vi "SaveDeviceHeader.vi"(0 "File Refnum in":refnum<file>, 1 "no. of arrays":i32, 3 "Array Lengths":i32, 5 "Filename":string, 7 "Run Number":i32, 9 "Array Titles":string, 11 "error in (no error)":errorcluster, 12 "Temperature":dbl, 13 "Humidity":dbl, 14 "Strip Segment":string) -> (4 "File Refnum out":refnum<file>, 6 "Header string":string, 10 "error out":errorcluster)   [LabVIEW 2018]
uses:
  globals/QC_RunInformation.vi
  globals/QC_MeasurementSetup.vi
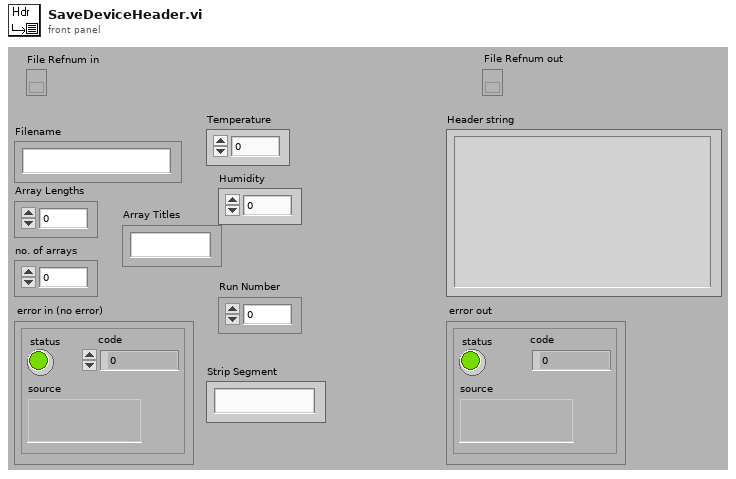
[diagram p1: front panel]
types:
  T1 = cluster{"Institute":string, "Manufacturers":string[], "Devices":string[], "Serialnumbers Lookup DB":string, "Data directory":string, "Backup & screenshot directory":string, "List of known users":string[], "Measurement switch not used":bool, "Measurement Switch":string, "DUT Switch":string}
  T2 = cluster{"Sensor Serial No.:":string, "Wafer Serial No.:":string, "Batch:":string, "Manufacturer:":string, "Device Category:":string, "Database Serial No.:":string, "Date Initiated:":string, "Time Initiated:":string, "Test":string, "Instruments used:":string, "Probeplan used:":string, "End of Run comment:":string, "User:":string}
  T3 = cluster{"Supply":refnum<class "SupplyControl.lvclass">, "LCR":refnum<class "LCRControl.lvclass">, "Initial Voltage [V]":dbl, "Final Voltage [V]":dbl, "Step Size [V]":dbl, "Step Interval [s]":i32, "Number Of Steps":u32, "AC frequency [Hz]":i32, "RC Configuration":u16, "AC amplitude [V]":dbl, "Ramp down steps [V]":dbl, "Ramp down Interval [s]":i32, "Set Current Limit?":bool, "Current Limit [µA]":dbl, "Temperature Readout":enum16{"Read Arduino", "Enter manually"}, "Arduino":refnum<class "ArduinoControl.lvclass">, "Supply Name":string, "LCR Name":string, "V_depletion Limit [V]":dbl, "Switching":refnum<class "Switching.lvclass">, "Matrix used?":bool, "Matrix X Channels":cluster{"Bias Supply / SMU LO":i32, "Bias Supply / SMU HI":i32, "CV Box LO":i32, "CV Box HI":i32, "CV Box LO IN":i32, "CV Box HI IN":i32, "Volt meter LO":i32, "Volt meter HI":i32, "Mux1 C1":i32, "Mux1 C2":i32, "Mux2 C1":i32, "Mux2 C2":i32}}
  T4 = cluster{"Bias Supply":refnum<class "SupplyControl.lvclass">, "SMU":refnum<class "SupplyControl.lvclass">, "LCR":refnum<class "LCRControl.lvclass">, "Probe Card Channels":i32, "Bias Voltage [V]":dbl, "First strip":i32, "Last strip":i32, "Base Voltage [V]":dbl, "Base Ramp Step [V]":dbl, "Base Ramp Interval [ms]":u32, "High Voltage [V]":dbl, "High Ramp Step [V]":dbl, "High Ramp Interval [ms]":u32, "AC frequency [Hz]":i32, "AC amplitude [V]":dbl, "RC Configuration":u16, "Single Needle":bool, "Temperature Readout":enum16{"Read Arduino", "Enter manually"}, "Arduino":refnum<class "ArduinoControl.lvclass">, "Fraction of good strips [%]":dbl, "ProbeStation":refnum<class "ProbeStationControl.lvclass">, "Switching":refnum<class "Switching.lvclass">, "Matrix used?":bool, "Matrix X Channels":cluster{"Bias Supply / SMU LO":i32, "Bias Supply / SMU HI":i32, "CV Box LO":i32, "CV Box HI":i32, "CV Box LO IN":i32, "CV Box HI IN":i32, "Volt meter LO":i32, "Volt meter HI":i32, "Mux1 C1":i32, "Mux1 C2":i32, "Mux2 C1":i32, "Mux2 C2":i32}, "Pinholes Y/N":bool, "Capacitance Y/N":bool, "Resistance Y/N":bool, "Bias Supply Name":string, "SMU Name":string, "LCR Name":string}
  T5 = cluster{"Supply":refnum<class "SupplyControl.lvclass">, "LCR":refnum<class "LCRControl.lvclass">, "Initial Voltage [V]":dbl, "Final Voltage [V]":dbl, "Step Size [V]":dbl, "Step Interval [s]":i32, "Number Of Steps":u32, "AC frequency [Hz]":i32, "RC Configuration":u16, "AC amplitude [V]":dbl, "Ramp down steps [V]":dbl, "Ramp down Interval [s]":i32, "Set Current Limit?":bool, "Current Limit [µA]":dbl, "Temperature Readout":enum16{"Read Arduino", "Enter manually"}, "Arduino":refnum<class "ArduinoControl.lvclass">, "Supply Name":string, "LCR Name":string, "C_is Limit [pF/cm]":dbl, "Switching":refnum<class "Switching.lvclass">, "Matrix used?":bool, "Matrix X Channels":cluster{"Bias Supply / SMU LO":i32, "Bias Supply / SMU HI":i32, "CV Box LO":i32, "CV Box HI":i32, "CV Box LO IN":i32, "CV Box HI IN":i32, "Volt meter LO":i32, "Volt meter HI":i32, "Mux1 C1":i32, "Mux1 C2":i32, "Mux2 C1":i32, "Mux2 C2":i32}}
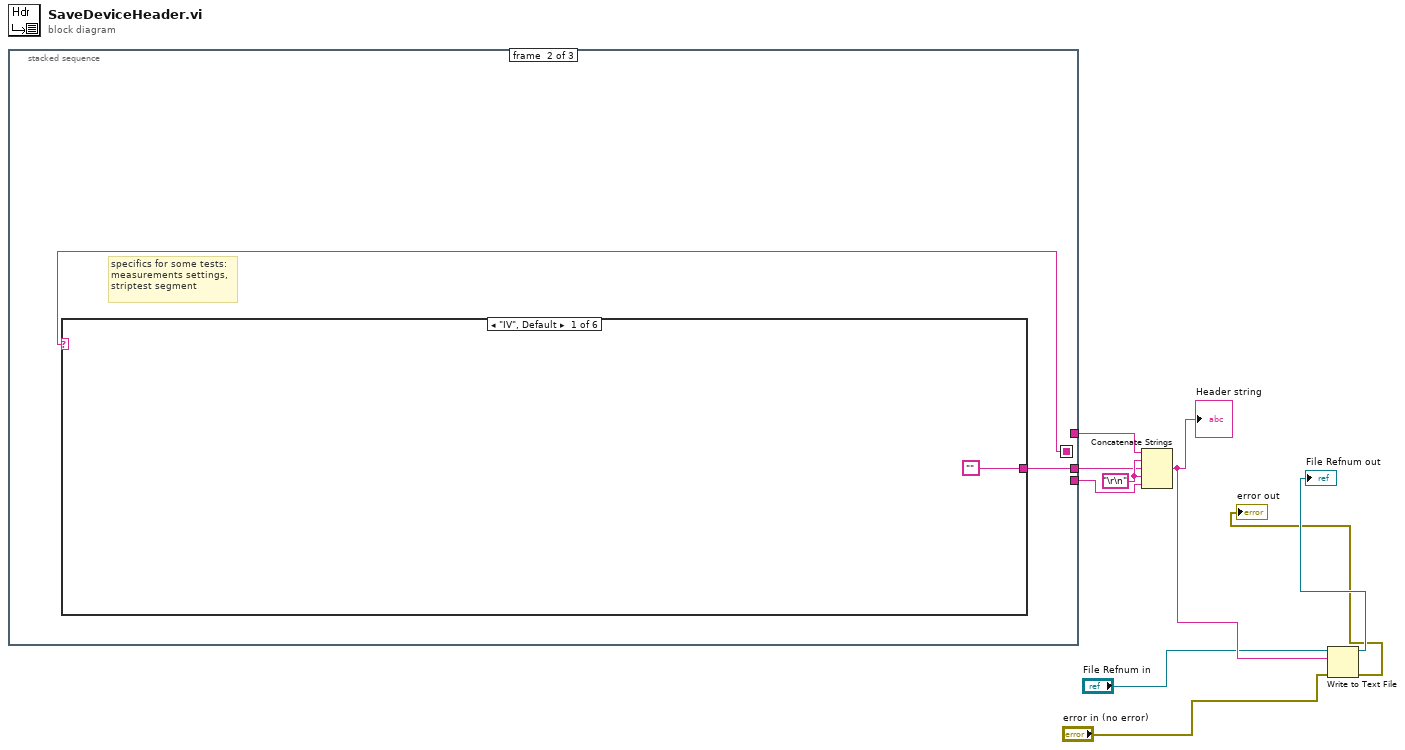
[diagram p0: block diagram]
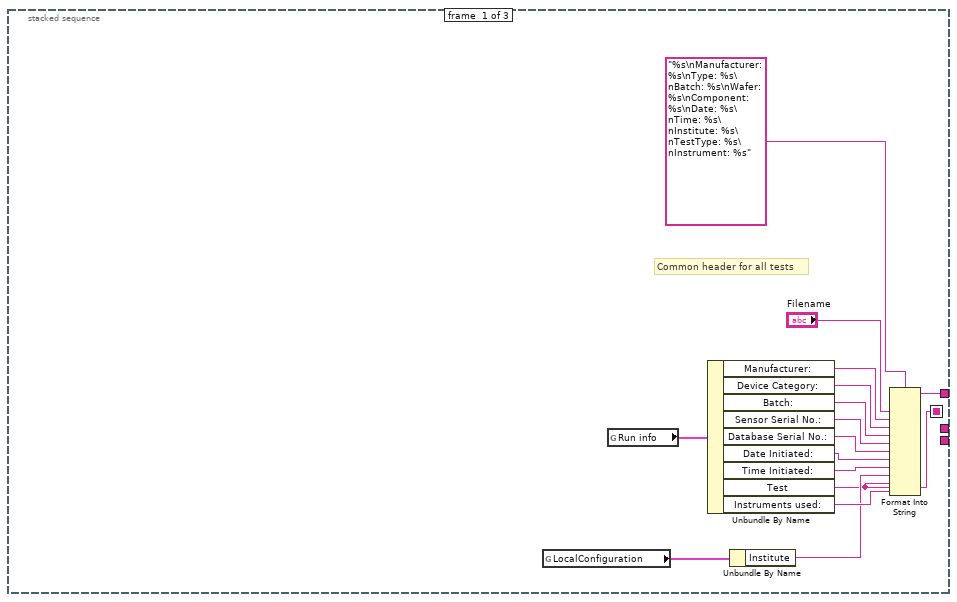
[diagram p2: hidden frame]
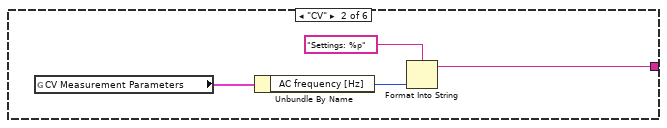
[diagram p3: hidden frame]
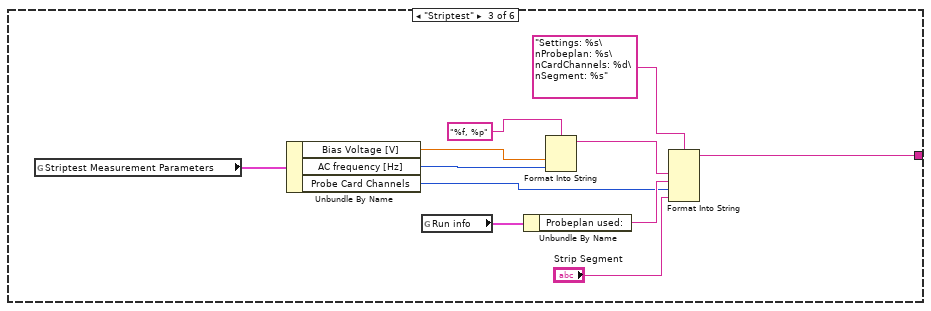
[diagram p4: hidden frame]
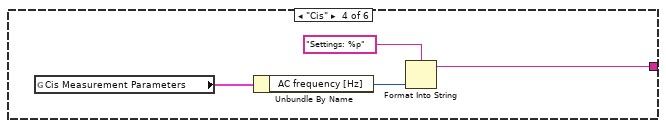
[diagram p5: hidden frame]
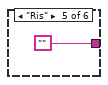
[diagram p6: hidden frame]
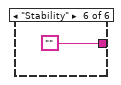
[diagram p7: hidden frame]
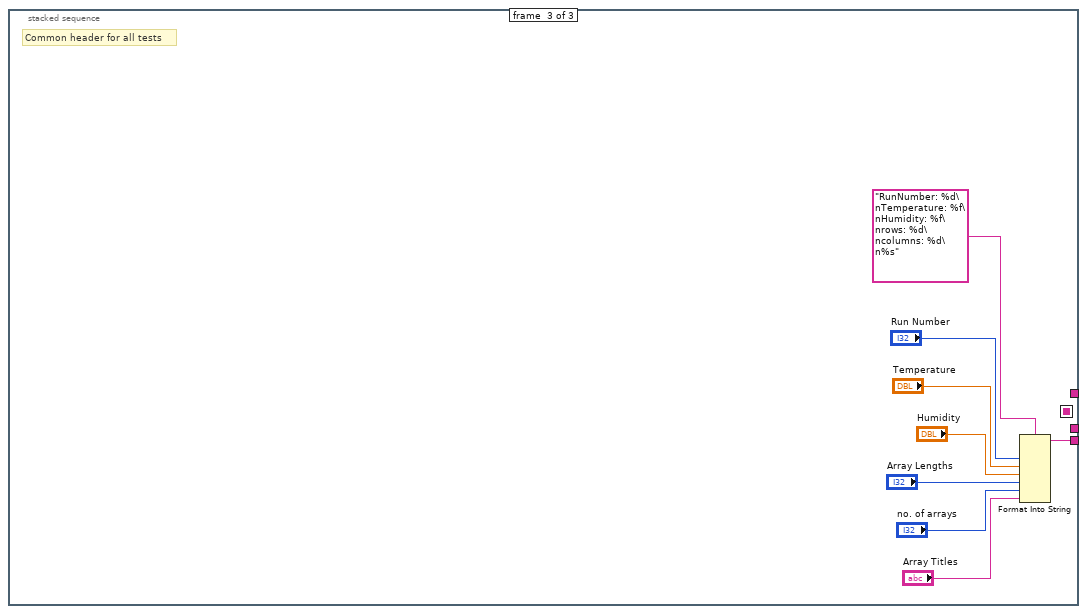
[diagram p8: hidden frame]
diagram:
  w9 = "\r\n"
  n1 = stacked-sequence {
    seq-local: [w11 _ _] -> [_ w26 _]
    tunnel: [_ w25 _] -> w8
    tunnel: [_ _ w49] -> w7
    tunnel: [w10 _ _] -> w6
    frame #0 {
      # "Common header for all tests"
      n2 = global read "QC_RunInformation.vi" "LocalConfiguration"() -> (w12:T1)
      n3 = global read "QC_RunInformation.vi" "Run info"() -> (w13:T2)
      n4 = Unbundle By Name(w13) -> ("Manufacturer:"=w15:string, "Device Category:"=w17:string, "Batch:"=w18:string, "Sensor Serial No.:"=w19:string, "Database Serial No.:"=w20:string, "Date Initiated:"=w21:string, "Time Initiated:"=w22:string, "Test"=w11:string, "Instruments used:"=w24:string)
      n5 = Unbundle By Name(w12) -> ("Institute"=w23:string)
      n6 = Format Into String(format string="%s\nManufacturer: %s\nType: %s\nBatch: %s\nWafer: %s\nComponent: %s\nDate: %s\nTime: %s\nInstitute: %s\nTestType: %s\nInstrument: %s", "Filename", w15, w17, w18, w19, w20, w21, w22, w23, w11, w24) -> (resulting string=w10:string)  [unwired: 2 in, 1 out]
    }
    frame #1 {
      # "specifics for some tests:\nmeasurements settings,\nstriptest segment"
      n7 = case shown="\"IV\", Default" w26 {
        tunnel: ["" w28 w33 w43 "" ""] -> w25
        frame "IV", Default {
        }
        frame "CV" {
          n8 = global read "QC_MeasurementSetup.vi" "CV Measurement Parameters"() -> (w29:T3)
          n9 = Unbundle By Name(w29) -> ("AC frequency [Hz]"=w31:i32)
          n10 = Format Into String(format string="Settings: %p", w31) -> (resulting string=w28:string)  [unwired: 2 in, 1 out]
        }
        frame "Striptest" {
          n11 = global read "QC_MeasurementSetup.vi" "Striptest Measurement Parameters"() -> (w41:T4)
          n12 = Unbundle By Name(w41) -> ("Bias Voltage [V]"=w38:dbl, "AC frequency [Hz]"=w37:i32, "Probe Card Channels"=w34:i32)
          n13 = global read "QC_RunInformation.vi" "Run info"() -> (w42:T2)
          n14 = Unbundle By Name(w42) -> ("Probeplan used:"=w35:string)
          n15 = Format Into String(format string="%f, %p", w38, w37) -> (resulting string=w36:string)  [unwired: 2 in, 1 out]
          n16 = Format Into String(format string="Settings: %s\nProbeplan: %s\nCardChannels: %d\nSegment: %s", w36, w35, w34, "Strip Segment") -> (resulting string=w33:string)  [unwired: 2 in, 1 out]
        }
        frame "Cis" {
          n17 = global read "QC_MeasurementSetup.vi" "Cis Measurement Parameters"() -> (w44:T5)
          n18 = Unbundle By Name(w44) -> ("AC frequency [Hz]"=w46:i32)
          n19 = Format Into String(format string="Settings: %p", w46) -> (resulting string=w43:string)  [unwired: 2 in, 1 out]
        }
        frame "Ris" {
        }
        frame "Stability" {
        }
      }
    }
    frame #2 {
      # "Common header for all tests"
      n20 = Format Into String(format string="RunNumber: %d\nTemperature: %f\nHumidity: %f\nrows: %d\ncolumns: %d\n%s", "Run Number", "Temperature", "Humidity", "Array Lengths", "no. of arrays", "Array Titles") -> (resulting string=w49:string)  [unwired: 2 in, 1 out]
    }
  }
  n21 = Concatenate Strings(w6, w9, w8, w9, w7) -> (w5:string)
  "Header string" <- w5
  n22 = Write to Text File(file (use dialog)="File Refnum in", text=w5, error in="error in (no error)") -> (refnum out=→"File Refnum out":refnum<file>, error out=→"error out":errorcluster)  [unwired: 1 in, 1 out]
